vi "VerifyChecksum.vi"(10 "String":string, 11 "ChecksumIndex":i32) -> (3 "ChecksumVerified":bool)   [LabVIEW 2014, in "Nav6.lvlib"]
uses:
  Nav6.lvlib
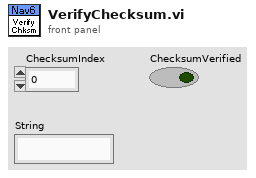
[diagram p1: front panel]
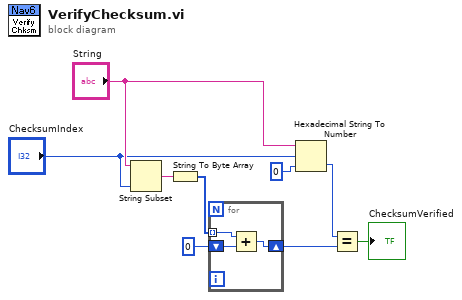
[diagram p0: block diagram]
diagram:
  n1 = String Subset(string="String", length (rest)="ChecksumIndex") -> (substring=w5:string)  [unwired: 1 in]
  n2 = String To Byte Array(string=w5) -> (unsigned byte array=w8:u8[])
  n3 = for {
    tunnel: w8 -> [w12] mode=indexing
    shift-right: [w11] -> w2
    shift-left: u8 0 -> [w10]
    n4 = Add(x=w12, y=w10) -> (x+y=w11:u8)
  }
  n5 = Hexadecimal String To Number(string="String", offset="ChecksumIndex", default (0uL)=u8 0 ("default (0 U32)")) -> (number=w3:u8)  [unwired: 1 out]
  n6 = Equal?(x=w3, y=w2) -> (x = y?=→"ChecksumVerified":bool)
